vi "S2DS_Timer.vi"(5 "Timer reset?":bool, 6 "WC read from file info (out)":T1, 7 "Scan parameters":T2 {"Y data taking" items=["in both direction", "in up direction only", "in down direction only"]; "X data taking" items=["in both direction", "in up direction only", "in down direction only"]}, 8 "Timer Cluster in":T3) -> (0 "Progress":i32, 1 "Remaining time":dbl, 2 "Elapsed time":dbl, 3 "Timer Cluster out":T3)   [LabVIEW 2025]
uses:
  TYPE DEFS/S2DS_Timer.ctl
  TYPE DEFS/S2DS_Sweep Info.ctl
  TYPE DEFS/S2DS_WCFromFileInfo.ctl
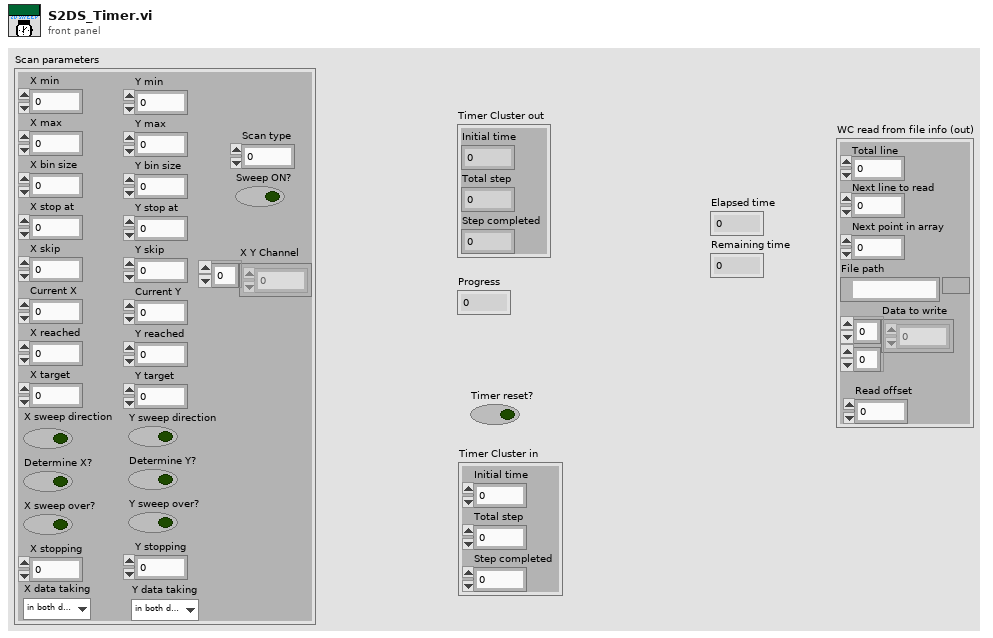
[diagram p1: front panel]
types:
  T1 = typedef "S2DS_WCFromFileInfo.ctl" = cluster{"Next line to read":i32, "Next point in array":i32, "File path":path, "Data to write":dbl[][], "Read offset":i32, "Total line":i32}
  T2 = typedef "S2DS_Sweep Info.ctl" = cluster{"X min":ext, "X max":dbl, "Y min":dbl, "Y max":dbl, "X bin size":dbl, "Y bin size":dbl, "X stop at":dbl, "Y stop at":dbl, "X skip":u64, "Y skip":u64, "Current X":dbl, "Current Y":dbl, "X reached":i32, "Y reached":i32, "X target":dbl, "Y target":dbl, "Sweep ON?":bool, "X sweep direction":bool, "Y sweep direction":bool, "Determine X?":bool, "Determine Y?":bool, "X sweep over?":bool, "Y sweep over?":bool, "Scan type":i32, "X stopping":i32, "Y stopping":i32, "X Y Channel":u16[], "X data taking":u16, "Y data taking":u16}
  T3 = typedef "S2DS_Timer.ctl" = cluster{"Initial time ":i32, "Total step":i32, "Step completed":i32}
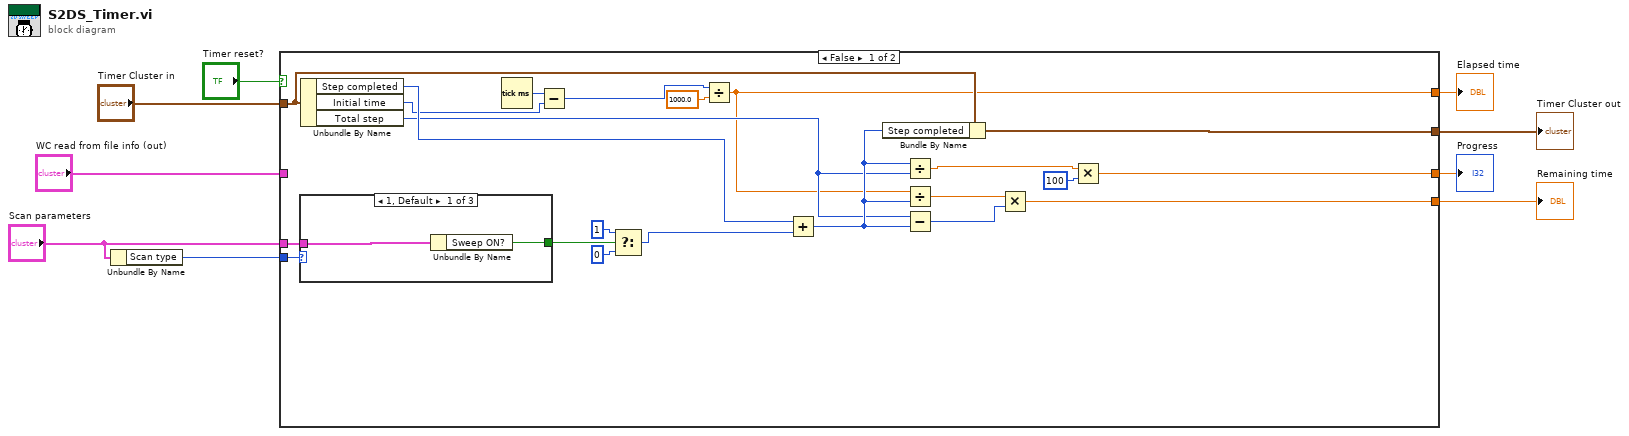
[diagram p0: block diagram]
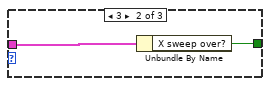
[diagram p2: hidden frame]
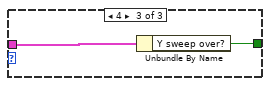
[diagram p3: hidden frame]
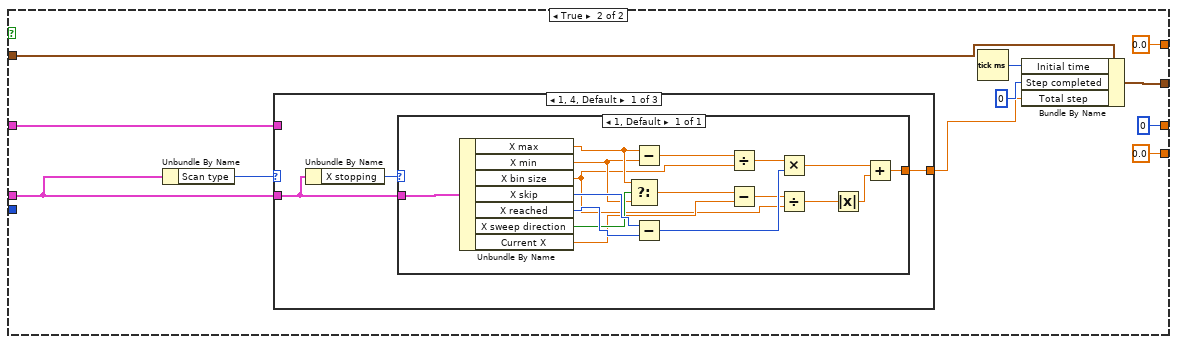
[diagram p4: hidden frame]
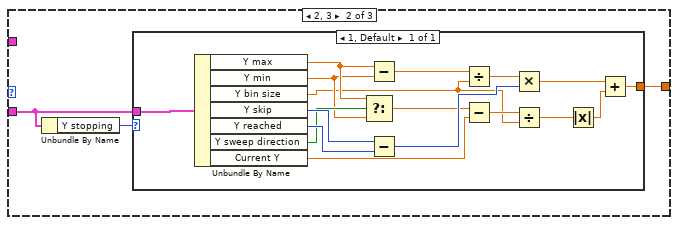
[diagram p5: hidden frame]
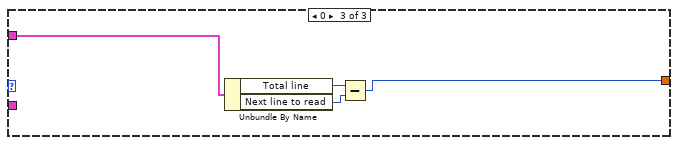
[diagram p6: hidden frame]
diagram:
  n1 = Unbundle By Name("Scan parameters") -> ("Scan type"=w5:i32)
  n2 = case shown="False" "Timer reset?" {
    tunnel: "Timer Cluster in" -> [w28 w48]
    tunnel: w5 -> [w15 _]
    tunnel: [w23 w45] -> w8
    tunnel: [w16 0] -> w9
    tunnel: "Scan parameters" -> [w14 w43]
    tunnel: [w12 0.0] -> w3
    tunnel: [w11 0.0] -> w2
    tunnel: "WC read from file info (out)" -> [_ w39]
    frame False {
      n3 = case shown="1, Default" w15 {
        tunnel: w14 -> [w33 w35 w37]
        tunnel: [w32 w34 w36] -> w13
        frame 1, Default {
          n4 = Unbundle By Name(w33) -> ("Sweep ON?"=w32:bool)
        }
        frame 3 {
          n5 = Unbundle By Name(w35) -> ("X sweep over?"=w34:bool)
        }
        frame 4 {
          n6 = Unbundle By Name(w37) -> ("Y sweep over?"=w36:bool)
        }
      }
      n7 = Unbundle By Name(w28) -> ("Step completed"=w29:i32, "Initial time"=w26:i32, "Total step"=w19:i32)
      n8 = Tick Count (ms)() -> (millisecond timer value=w27:u32)
      n9 = Subtract(x=w27, y=w26) -> (x-y=w24:u32)
      n10 = Select(t=1, s=w13, f=0) -> (s? t:f=w10:i32)
      n11 = Divide(x=w24, y=1000.0) -> (x/y=w12:dbl)
      n12 = Add(x=w29, y=w10) -> (x+y=w20:i32)
      n13 = Bundle By Name(cluster=w28, "Step completed"=w20) -> (w23:T3)
      n14 = Divide(x=w20, y=w19) -> (x/y=w18:dbl)
      n15 = Divide(x=w12, y=w20) -> (x/y=w22:dbl)
      n16 = Subtract(x=w19, y=w20) -> (x-y=w21:i32)
      n17 = Multiply(x=w22, y=w21) -> (x*y=w11:dbl)
      n18 = Multiply(x=w18, y=100) -> (x*y=w16:dbl)
    }
    frame True {
      n19 = Unbundle By Name(w43) -> ("Scan type"=w38:i32)
      n20 = case shown="1, 4, Default" w38 {
        tunnel: w43 -> [w51 w71 _]
        tunnel: [w49 w69 w90] -> w42
        tunnel: w39 -> [_ _ w89]
        frame 1, 4, Default {
          n21 = Unbundle By Name(w51) -> ("X stopping"=w50:i32)
          n22 = case shown="1, Default" w50 {
            tunnel: w51 -> [w68]
            tunnel: [w52] -> w49
            frame 1, Default {
              n23 = Unbundle By Name(w68) -> ("X max"=w61:dbl, "X min"=w60:ext, "X bin size"=w56:dbl, "X skip"=w66:u64, "X reached"=w65:i32, "X sweep direction"=w62:bool, "Current X"=w58:dbl)
              n24 = Select(t=w61, s=w62, f=w60) -> (s? t:f=w59:ext)
              n25 = Subtract(x=w61, y=w60) -> (x-y=w67:ext)
              n26 = Subtract(x=w66, y=w65) -> (x-y=w63:u64)
              n27 = Divide(x=w67, y=w56) -> (x/y=w64:ext)
              n28 = Subtract(x=w59, y=w58) -> (x-y=w57:ext)
              n29 = Multiply(x=w64, y=w63) -> (x*y=w53:ext)
              n30 = Divide(x=w57, y=w56) -> (x/y=w55:ext)
              n31 = Absolute Value(x=w55) -> (abs(x)=w54:ext)
              n32 = Add(x=w53, y=w54) -> (x+y=w52:ext)
            }
          }
        }
        frame 2, 3 {
          n33 = Unbundle By Name(w71) -> ("Y stopping"=w70:i32)
          n34 = case shown="1, Default" w70 {
            tunnel: w71 -> [w88]
            tunnel: [w72] -> w69
            frame 1, Default {
              n35 = Unbundle By Name(w88) -> ("Y max"=w81:dbl, "Y min"=w80:dbl, "Y bin size"=w76:dbl, "Y skip"=w86:u64, "Y reached"=w85:i32, "Y sweep direction"=w82:bool, "Current Y"=w78:dbl)
              n36 = Select(t=w81, s=w82, f=w80) -> (s? t:f=w79:dbl)
              n37 = Subtract(x=w81, y=w80) -> (x-y=w87:dbl)
              n38 = Subtract(x=w86, y=w85) -> (x-y=w83:u64)
              n39 = Divide(x=w87, y=w76) -> (x/y=w84:dbl)
              n40 = Subtract(x=w79, y=w78) -> (x-y=w77:dbl)
              n41 = Multiply(x=w84, y=w83) -> (x*y=w73:dbl)
              n42 = Divide(x=w77, y=w76) -> (x/y=w75:dbl)
              n43 = Absolute Value(x=w75) -> (abs(x)=w74:dbl)
              n44 = Add(x=w73, y=w74) -> (x+y=w72:dbl)
            }
          }
        }
        frame 0 {
          n45 = Unbundle By Name(w89) -> ("Total line"=w92:i32, "Next line to read"=w91:i32)
          n46 = Subtract(x=w92, y=w91) -> (x-y=w90:i32)
        }
      }
      n47 = Tick Count (ms)() -> (millisecond timer value=w47:u32)
      n48 = Bundle By Name(cluster=w48, "Initial time"=w47, "Step completed"=0, "Total step"=w42) -> (w45:T3)
    }
  }
  "Progress" <- w9
  "Timer Cluster out" <- w8
  "Elapsed time" <- w3
  "Remaining time" <- w2
